vi "Backing up cost.vi"(10 "Resolution":i32=200, 11 "Scale":dbl=0.1) -> (3 "Intensity Graph":dbl[][](graph))   [LabVIEW 2012]
uses:
  <vilib>/imath/engines/lvmath2/RunTimeEngine/ErrorHandling/NIMS_Finalize Error.vi
  <vilib>/imath/engines/lvmath2/RunTimeEngine/Managers/WorkSpace/UID Generator.vi
  <vilib>/imath/engines/lvmath2/RunTimeEngine/Managers/SymbolTable/Clear UID.vi
  <vilib>/imath/engines/lvmath2/RunTimeEngine/NodeEndStatement/NIMS_NodeEndStatement_Output.vi
  <instcachedir>/0/NIMS_NodeEndStatement_Output_53EC0D466D134D7ABD903AC30B43404B.lvgen/NIMS_NodeEndStatement_Output_53EC0D466D134D7ABD903AC30B43404B_001.vi
  <vilib>/imath/engines/lvmath2/RunTimeEngine/RunTimeType/NIMS_RunTimeType_From StrictType (excl LVString).vi
  <instcachedir>/0/NIMS_RunTimeType_From StrictType (excl LVString)_AC52D965D0864706932D20A05968E122.lvgen/NIMS_RunTimeType_From StrictType (excl LVString)_AC52D965D0864706932D20A05968E122_000.vi
  <vilib>/imath/engines/lvmath2/RunTimeEngine/LocalVariableDefStatement/MC_LocalVariableDefStatement_Display.vi
  <vilib>/Analysis/1siggen.llb/Ramp Pattern by Samples.vi
  <vilib>/Analysis/NI_AALBase.lvlib
  <vilib>/imath/engines/lvmath2/RunTimeEngine/Managers/SymbolTable/NIMS_WorkSpace.lvlib
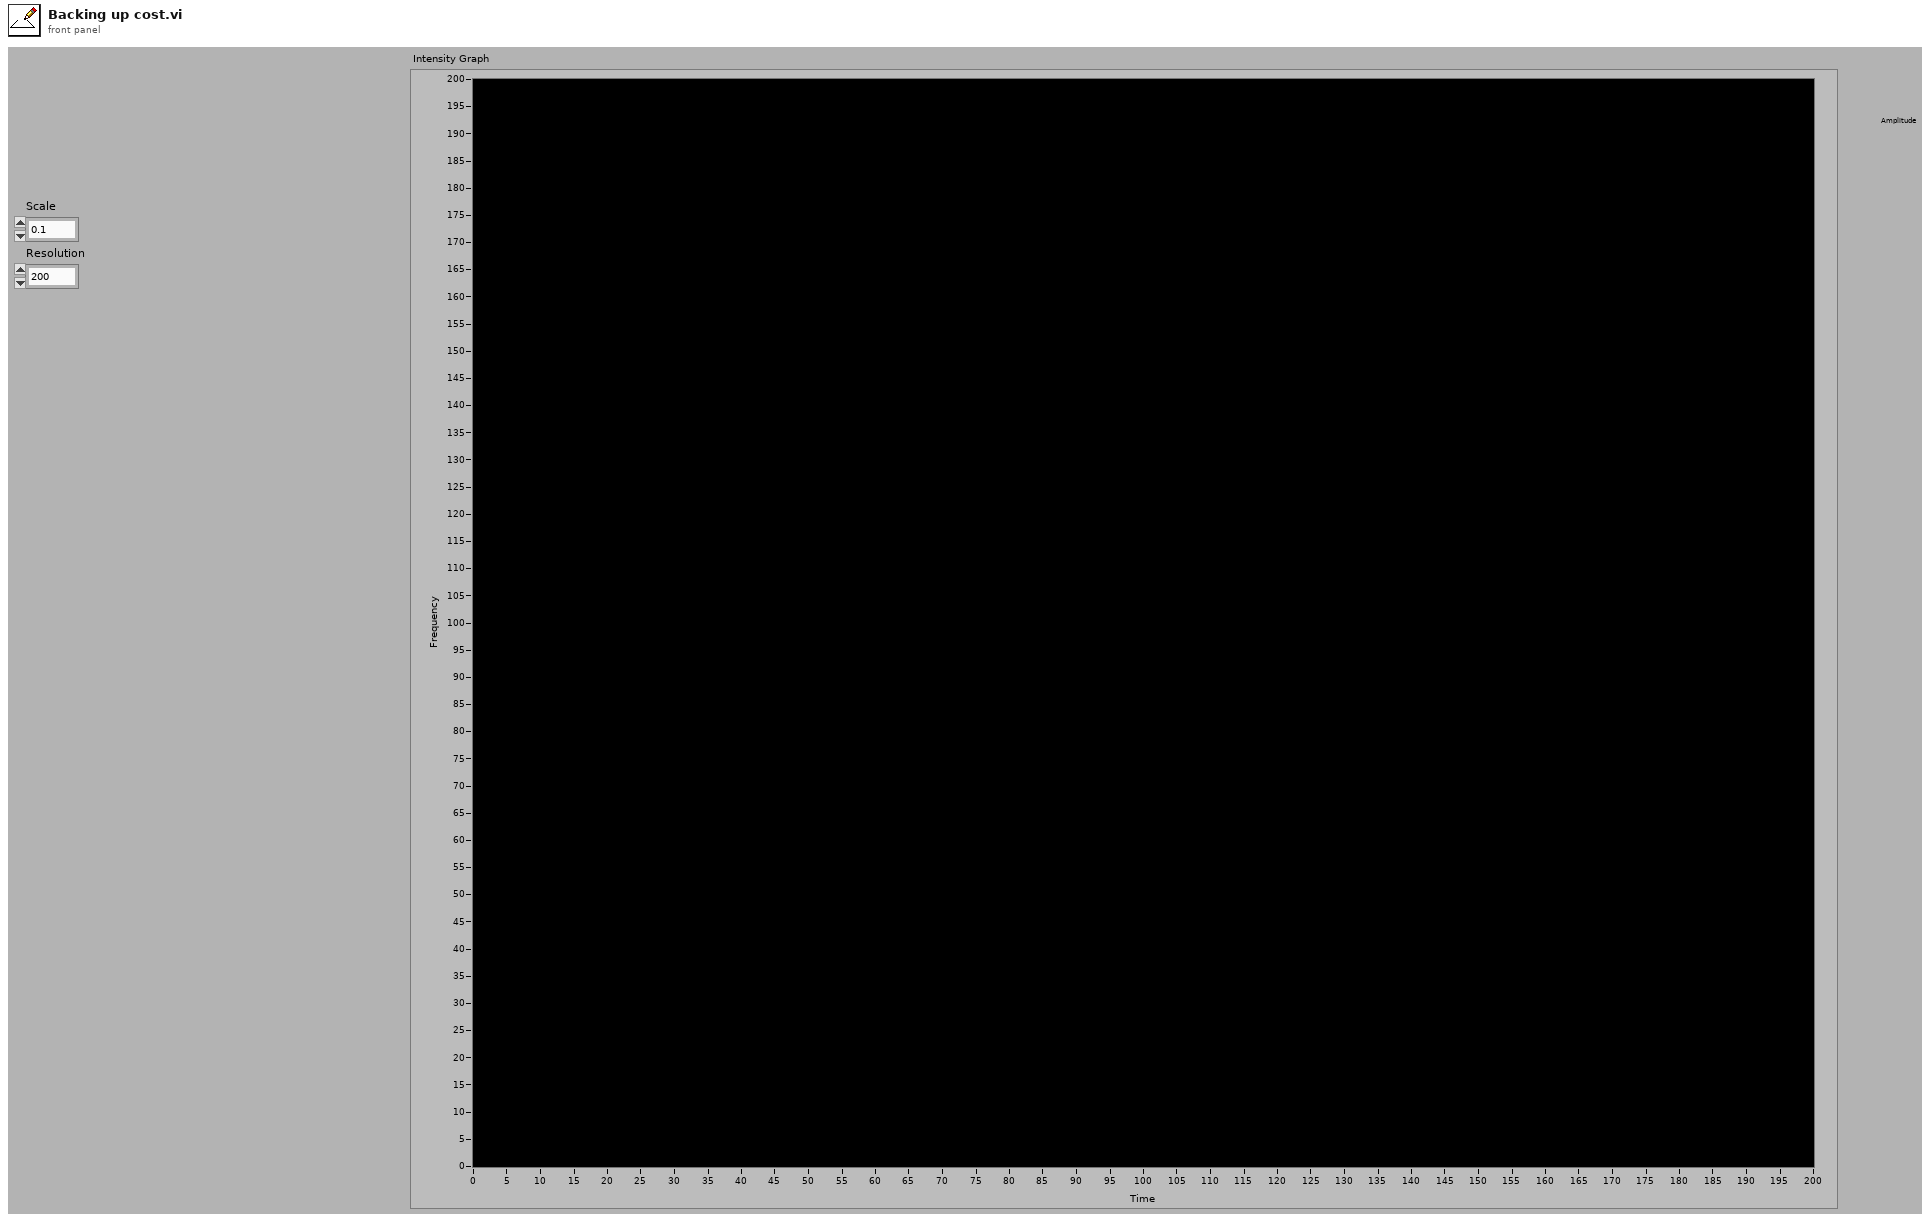
[diagram p1: front panel]
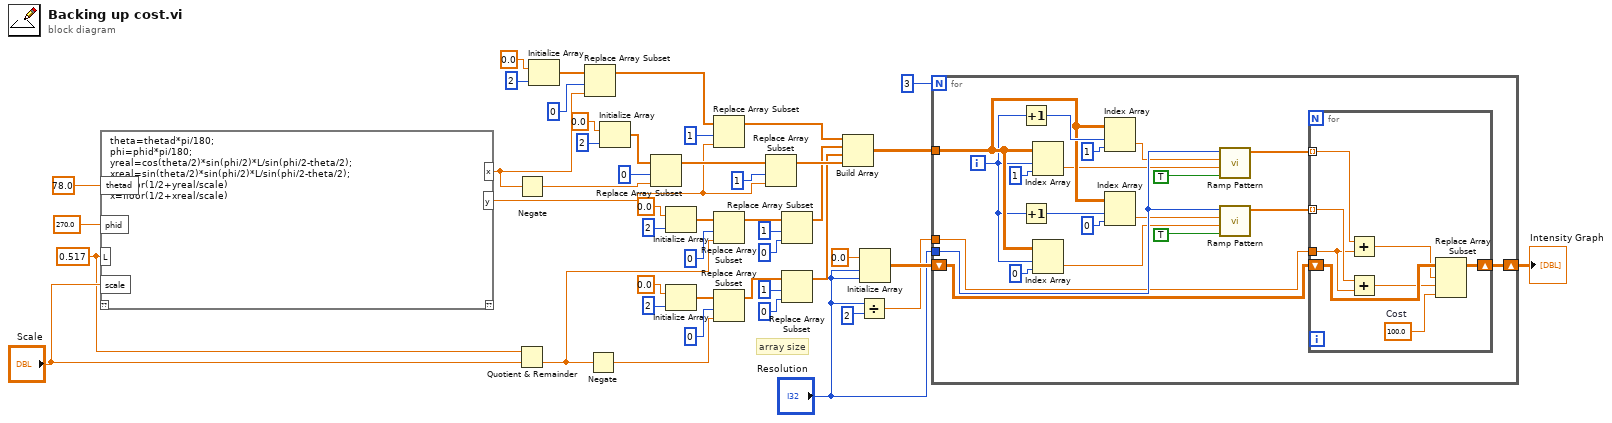
[diagram p0: block diagram]
diagram:
  w1 = 0.517
  # "array size"
  n1 = mathscript code="theta=thetad*pi/180;\nphi=phid*pi/180;\nyreal=cos(theta/2)*sin(phi/2)*L/sin(phi/2-theta/2);\nxreal=sin(theta/2)*sin(phi/2)*L/sin(phi/2-theta/2);\ny=floor(1/2+yreal/scale)\nx=floor(1/2+xreal/scale)"("L"=w1, "thetad"=78.0 ("theta"), "phid"=270.0, "scale"="Scale") -> ("x"=w27:dbl, "y"=w30:dbl)  [unwired: 1 in, 1 out]
  n2 = Negate(x=w27) -> (-x=w28:dbl)
  n3 = Quotient & Remainder(x=w1, y="Scale") -> (floor(x/y)=w10:dbl)  [unwired: 1 out]
  n4 = Initialize Array(0.0 ("element"), 2 ("dimension size")) -> (w41:dbl[])
  n5 = Replace Array Subset(array=w41, new element=w27, index=0) -> (w39:dbl[])
  n6 = Negate(x=w10) -> (-x=w11:dbl)
  n7 = Initialize Array(0.0 ("element"), 2 ("dimension size")) -> (w35:dbl[])
  n8 = Replace Array Subset(array=w35, new element=w28, index=0) -> (w33:dbl[])
  n9 = Initialize Array(0.0 ("element"), 2 ("dimension size")) -> (w24:dbl[])
  n10 = Initialize Array(0.0 ("element"), 2 ("dimension size")) -> (w17:dbl[])
  n11 = Replace Array Subset(array=w39, new element=w30, index=1) -> (w36:dbl[])
  n12 = Replace Array Subset(array=w24, new element=w10, index=0) -> (w22:dbl[])
  n13 = Replace Array Subset(array=w17, new element=w11, index=0) -> (w15:dbl[])
  n14 = Replace Array Subset(array=w33, new element=w30, index=1) -> (w26:dbl[])
  n15 = Replace Array Subset(array=w22, new element=0 ("index"), index=1) -> (w19:dbl[])
  n16 = Replace Array Subset(array=w15, new element=0 ("index"), index=1) -> (w12:dbl[])
  n17 = Build Array(w36, w19, w12, w26) -> (w7:dbl[][])
  n18 = Divide(x="Resolution", y=2) -> (x/y=w2:dbl)
  n19 = Initialize Array(0.0 ("element"), "Resolution", "Resolution") -> (w46:dbl[][])
  n20 = for {
    N: 3 -> [_]
    tunnel: "Resolution" -> [w67]
    shift-right: [w64] -> w6
    shift-left: w46 -> [w63]
    tunnel: w7 -> [w53]
    tunnel: w2 -> [w48]
    i -> [w52]
    n21 = Increment(x=w52) -> (x+1=w55:i32)
    n22 = Increment(x=w52) -> (x+1=w60:i32)
    n23 = Index Array(array=w53, index (row)=w52, index (col)=1 ("disabled index (col)")) -> (element=w51:dbl)
    n24 = Index Array(array=w53, index (row)=w52, index (col)=0 ("disabled index (col)")) -> (element=w62:dbl)
    n25 = Index Array(array=w53, index (row)=w55, index (col)=1 ("disabled index (col)")) -> (element=w50:dbl)
    n26 = Index Array(array=w53, index (row)=w60, index (col)=0 ("disabled index (col)")) -> (element=w58:dbl)
    n27 = call-poly <vilib>:"Ramp Pattern.vi"("exclude end?"=TRUE, "start"=w51, "end"=w50, "samples"=w67) -> ("Ramp Pattern"=w65:dbl[])  [unwired: 6 in, 1 out]
    n28 = call-poly <vilib>:"Ramp Pattern.vi"("exclude end?"=TRUE, "start"=w62, "end"=w58, "samples"=w67) -> ("Ramp Pattern"=w66:dbl[])  [unwired: 6 in, 1 out]
    n29 = for {
      tunnel: w66 -> [w71] mode=indexing
      tunnel: w65 -> [w72] mode=indexing
      shift-right: [w73] -> w64
      shift-left: w63 -> [w74]
      tunnel: w48 -> [w70]
      w75 = 100.0  # Cost
      n30 = Add(x=w72, y=w70) -> (x+y=w68:dbl)
      n31 = Add(x=w71, y=w70) -> (x+y=w69:dbl)
      n32 = Replace Array Subset(array=w74, new element=w75, index (row)=w68, index (col)=w69) -> (w73:dbl[][])
    }
  }
  "Intensity Graph" <- w6
